vi "VI Server_TREE_ActiveCell_Font_SET.vi"(4 "Cluster":T1, 6 "AciveCell.Position":T2={"Row Number\n(-2-all clmns)"=0, "Column Number\n(-2 - whole row)"=3} {"Column Number\n(-2 - whole row)" min=-2}, 7 "Label":string, 8 "error in":errorcluster, 9 "Tree.Ref":refnum<vi>, 10 "SingleInstance":bool=TRUE, 11 "VI Server.RefsCluster":T3) -> (0 "error out":errorcluster, 1 "Tree.Ref.DUP":refnum<vi>, 3 "VI Server.RefsCluster.DUP":T3)   [LabVIEW 2020]
uses:
  VI Server_TypeDefs/VI Server_RefsCluster.ctl
  VI Server_TypeDefs/VI Server_TREE_ActiveCell_Pos.ctl
  <vilib>/Utility/miscctls.llb/LVFontTypeDef.ctl
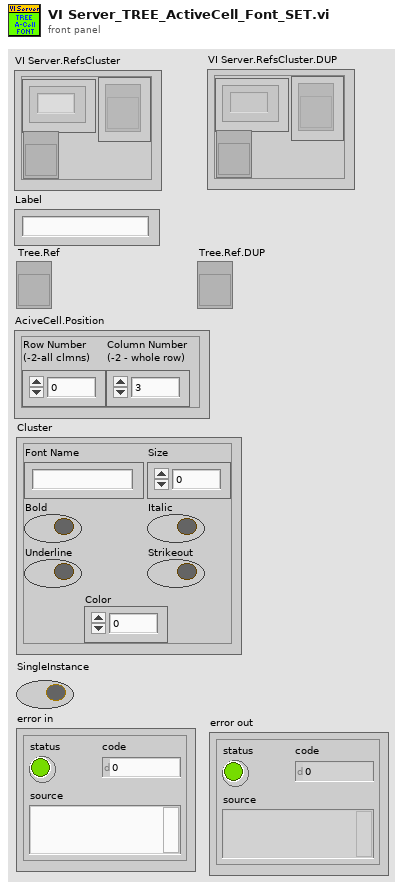
[diagram p1: front panel]
types:
  T1 = cluster{"Font Name":string, "Size":u16, "Bold":bool, "Italic":bool, "Underline":bool, "Strikeout":bool, "Color":u32}
  T2 = typedef "VI Server_TREE_ActiveCell_Pos.ctl" = cluster{"Row Number\n(-2-all clmns)":i32, "Column Number\n(-2 - whole row)":i32}
  T3 = typedef "VI Server_RefsCluster.ctl" = cluster{"Labels":string[], "Refs":refnum<vi>[], "VI Ref":refnum<vi>}
  T4 = typedef "LVFontTypeDef.ctl" = cluster{"Font Name":string, "Size":u16, "Bold":bool, "Italic":bool, "Underline":bool, "Strikeout":bool, "Color":u32}
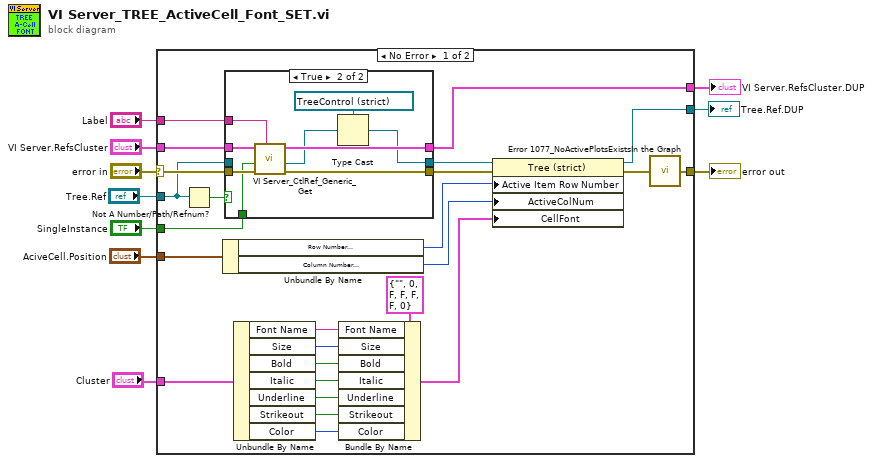
[diagram p0: block diagram]
diagram:
  n1 = case shown="No Error" "error in" {
    selector: "error in" -> [w35 w49]
    tunnel: [w11 w49] -> w9
    tunnel: "VI Server.RefsCluster" -> [w34 w48]
    tunnel: [w33 w48] -> w7
    tunnel: "Label" -> [w32 _]
    tunnel: "SingleInstance" -> [w31 _]
    tunnel: [w26 _] -> w1
    tunnel: "Tree.Ref" -> [w29 _]
    tunnel: "AciveCell.Position" -> [w25 _]
    tunnel: "Cluster" -> [w21 _]
    frame No Error {
      n2 = Not A Number/Path/Refnum?(number/path/refnum=w29) -> (NaN/Path/Refnum?=w30:bool)
      n3 = Unbundle By Name(w25) -> ("Row Number\n(-2-all clmns)"=w24:i32, "Column Number\n(-2 - whole row)"=w23:i32)
      n4 = case shown="True" w30 {
        tunnel: w35 -> [w38 w47]
        tunnel: w34 -> [w36 w46]
        tunnel: [w36 w45] -> w33
        tunnel: w32 -> [_ w44]
        tunnel: w31 -> [_ w42]
        tunnel: [w37 w41] -> w28
        tunnel: [w38 w40] -> w27
        tunnel: w29 -> [w37 _]
        frame False {
        }
        frame True {
          n5 = call "VI Server_CtlRef_Generic_Get.vi"("Control.Label"=w44, "error in"=w47, "SingleInstance"=w42, "VI Server.RefsCluster"=w46) -> ("error out"=w40:errorcluster, "Control.Ref.Generic"=w43:refnum<vi>, "VI Server.RefsCluster.DUP"=w45:T3)  [unwired: 5 in]
          n6 = Type Cast(type=refnum<vi> refnum ("Test.Tree"), x=w43) -> (*(type *) &x=w41:refnum<vi>)
        }
      }
      n7 = Unbundle By Name(w21) -> ("Font Name"=w20:string, "Size"=w19:u16, "Bold"=w18:bool, "Italic"=w17:bool, "Underline"=w16:bool, "Strikeout"=w15:bool, "Color"=w14:u32)
      n8 = Bundle By Name(cluster=T4 {"Font Name"="", "Size"=0, "Bold"=FALSE, "Italic"=FALSE, "Underline"=FALSE, "Strikeout"=FALSE, "Color"=0} ("Active Cell:Cell Font"), "Font Name"=w20, "Size"=w19, "Bold"=w18, "Italic"=w17, "Underline"=w16, "Strikeout"=w15, "Color"=w14) -> (w13:T4)
      n9 = property on="Property Node" class="Tree (strict)"(reference=w28, error in=w27, "Active Item Row Number"=w24, "ActiveColNum"=w23, "CellFont"=w13) -> (reference out=w26:refnum<vi>, error out=w12:errorcluster)
      n10 = call "Error 1077_NoActivePlotsExistsIn the Graph.vi"("error in"=w12) -> ("error out"=w11:errorcluster)  [unwired: 4 in]
    }
    frame Error {
    }
  }
  "VI Server.RefsCluster.DUP" <- w7
  "error out" <- w9
  "Tree.Ref.DUP" <- w1
